vi "subvi Robot Extract ROI Info.vi"(0 "ROIListBoxIn":string[][](array[string]), 1 "Selection":i32) -> (2 "ROIName":string, 3 "TotalTiles":u32, 4 "XYListOffset":u32, 5 "TileSuffix":string[](array[string]))   [LabVIEW 2012]
panel:
  out "TileY":u32
  out "TileX":u32
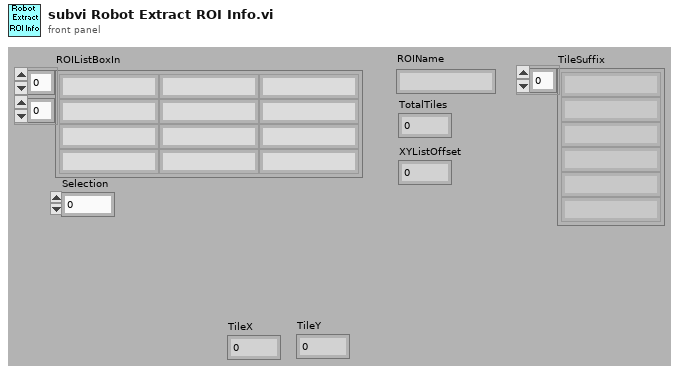
[diagram p1: front panel]
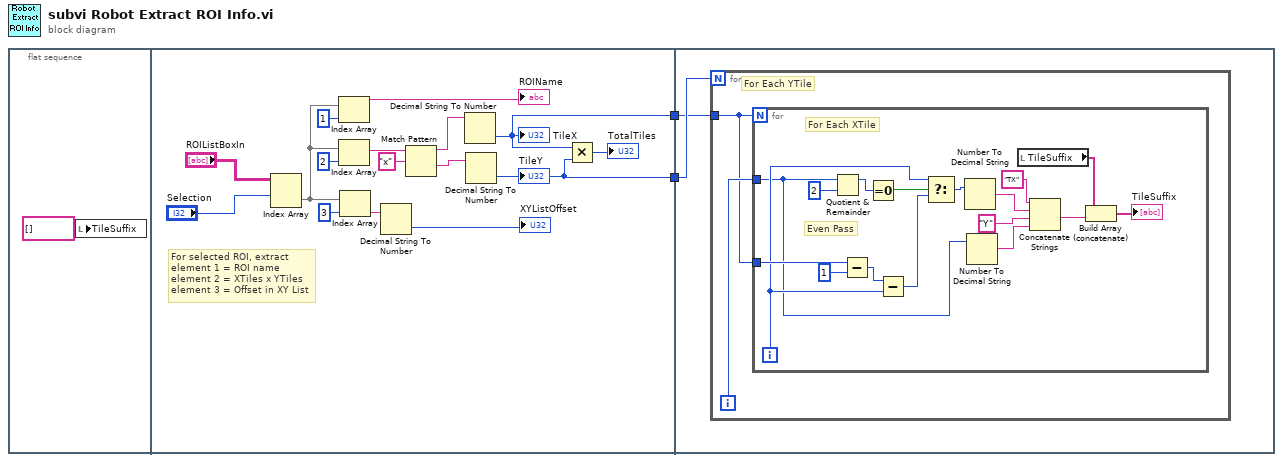
[diagram p0: block diagram]
diagram:
  n1 = flat-sequence {
    tunnel: [w6] -> w2
    tunnel: [w5] -> w1
    tunnel: w2 -> [w21]
    tunnel: w1 -> [w20]
    frame #0 {
      n2 = local write "TileSuffix"(string[] [] ("TileSuffix")) -> ()
    }
    frame #1 {
      # "For selected ROI, extract\nelement 1 = ROI name\nelement 2 = XTiles x YTiles\nelement 3 = Offset in XY List"
      n3 = Index Array(array="ROIListBoxIn", index (row)="Selection") -> (element=w10:string[])  [unwired: 1 in]
      n4 = Index Array(array=w10, index=1) -> (element=→"ROIName":string)
      n5 = Index Array(array=w10, index=2) -> (element=w14:string)
      n6 = Index Array(array=w10, index=3) -> (element=w9:string)
      n7 = Decimal String To Number(string=w9) -> (number=→"XYListOffset":i32)  [unwired: 3 out]
      n8 = Match Pattern(string=w14, regular expression="x") -> (before substring=w13:string, after substring=w12:string)  [unwired: 3 out]
      n9 = Decimal String To Number(string=w13) -> (number=w5:i32)  [unwired: 3 out]
      "TileX" <- w5
      n10 = Decimal String To Number(string=w12) -> (number=w6:i32)  [unwired: 3 out]
      "TileY" <- w6
      n11 = Multiply(x=w5, y=w6) -> (x*y=→"TotalTiles":i32)
    }
    frame #2 {
      n12 = for {
        N: w21 -> [_]
        tunnel: w20 -> [w22]
        i -> [w23]
        # "For Each YTile"
        n13 = for {
          N: w22 -> [_]
          tunnel: w23 -> [w26]
          tunnel: w22 -> [w33]
          i -> [w31]
          # "For Each XTile"
          # "Even Pass"
          n14 = Quotient & Remainder(x=w26, y=2) -> (x-y*floor(x/y)=w35:i32)  [unwired: 1 out]
          n15 = Subtract(x=w33, y=u32 1) -> (x-y=w37:u32)
          n16 = Equal To 0?(x=w35) -> (x = 0?=w39:bool)
          n17 = Subtract(x=w37, y=w31) -> (x-y=w36:u32)
          n18 = Select(t=w31, s=w39, f=w36) -> (s? t:f=w32:u32)
          n19 = Number To Decimal String(number=w32) -> (decimal integer string=w34:string)  [unwired: 1 out]
          n20 = Number To Decimal String(number=w26) -> (decimal integer string=w25:string)  [unwired: 1 out]
          n21 = local read "TileSuffix"() -> (w30:string[])
          n22 = Concatenate Strings("TX" ("string"), w34, "Y" ("string"), w25) -> (w28:string)
          n23 = Build Array (concatenate)(w30, w28) -> (→"TileSuffix":string[])
        }
      }
    }
  }
